vi "数据查询_仪器数据.vi"() -> ()   [LabVIEW 2016, in "数据查询.lvlib"]
uses:
  <vilib>/Utility/miscctls.llb/LVPointTypeDef.ctl
  <vilib>/Utility/miscctls.llb/LVRowAndColumnUnsignedTypeDef.ctl
  <userlib>/_OpenG.lib/array/array.llb/Sort 2D Array (String)__ogtk.vi
  <vilib>/ptbypt/NI_PtbyPt.lvlib
panel:
  out "布尔":bool=TRUE
  in  "显示关键参数":bool
  in  "剔除异常数据":bool
  in  "数据类型":string(combo)="全部数据"
  in  "列表框":i32(listbox)
  in  "页":i32 format="第%.0f页"
  in  "每页条数":i32=1000
  in  "向后按钮":bool
  in  "向前按钮":bool
  in  "导出":bool
  in  "测量模式":string(combo)="全部数据"
  in  "查询":bool
  in  "结束日期":string="2050/01/01"
  in  "起始日期":string="2010/01/01"
  out "数据表":string[][](table)
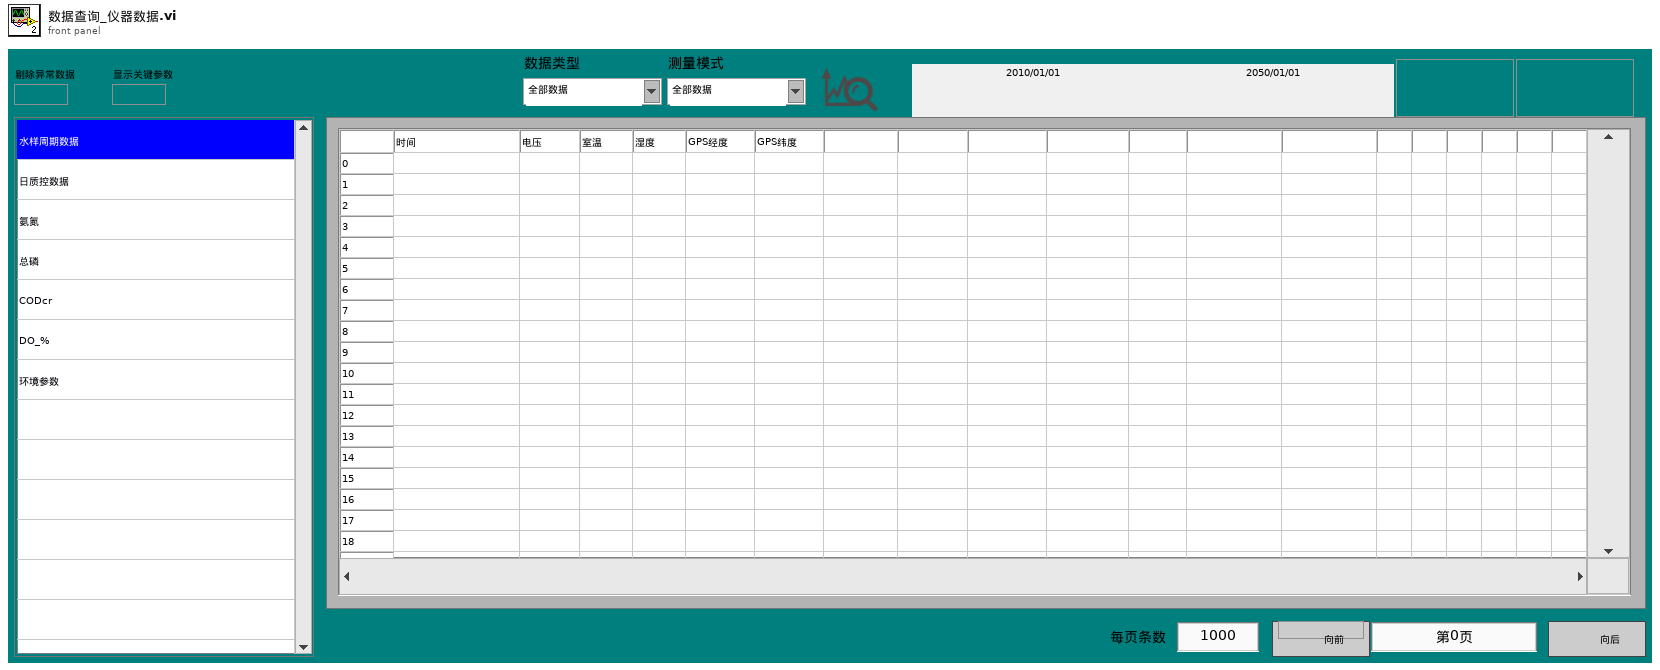
[diagram p1: front panel]
types:
  T1 = typedef "LVPointTypeDef.ctl" = cluster{"Horizontal":i16, "Vertical":i16}
  T2 = typedef "LVDateTimeRec.ctl" = cluster{"秒数的小数部分":dbl, "秒":i32, "分":i32, "时":i32, "日":i32, "月":i32, "年":i32, "天数（周）":i32, "天数（年）":i32, "DST":i32}
  T3 = typedef "Rendezvous RefNum" = refnum<k1>
  T4 = typedef "数据查询.lvlib/数据查询单选控件.ctl" = enum32{"数据查询", "仪器数据", "仪器日志", "报警信息", "校准日志"}
  T5 = enum8{"Enabled", "Disabled", "Disabled and Grayed Out"}
  T6 = typedef "LVRowAndColumnUnsignedTypeDef.ctl" = cluster{"Row":u32, "Column":u32}
  T7 = typedef "数据库类型.ctl" = enum16{"Access", "SQLite"}
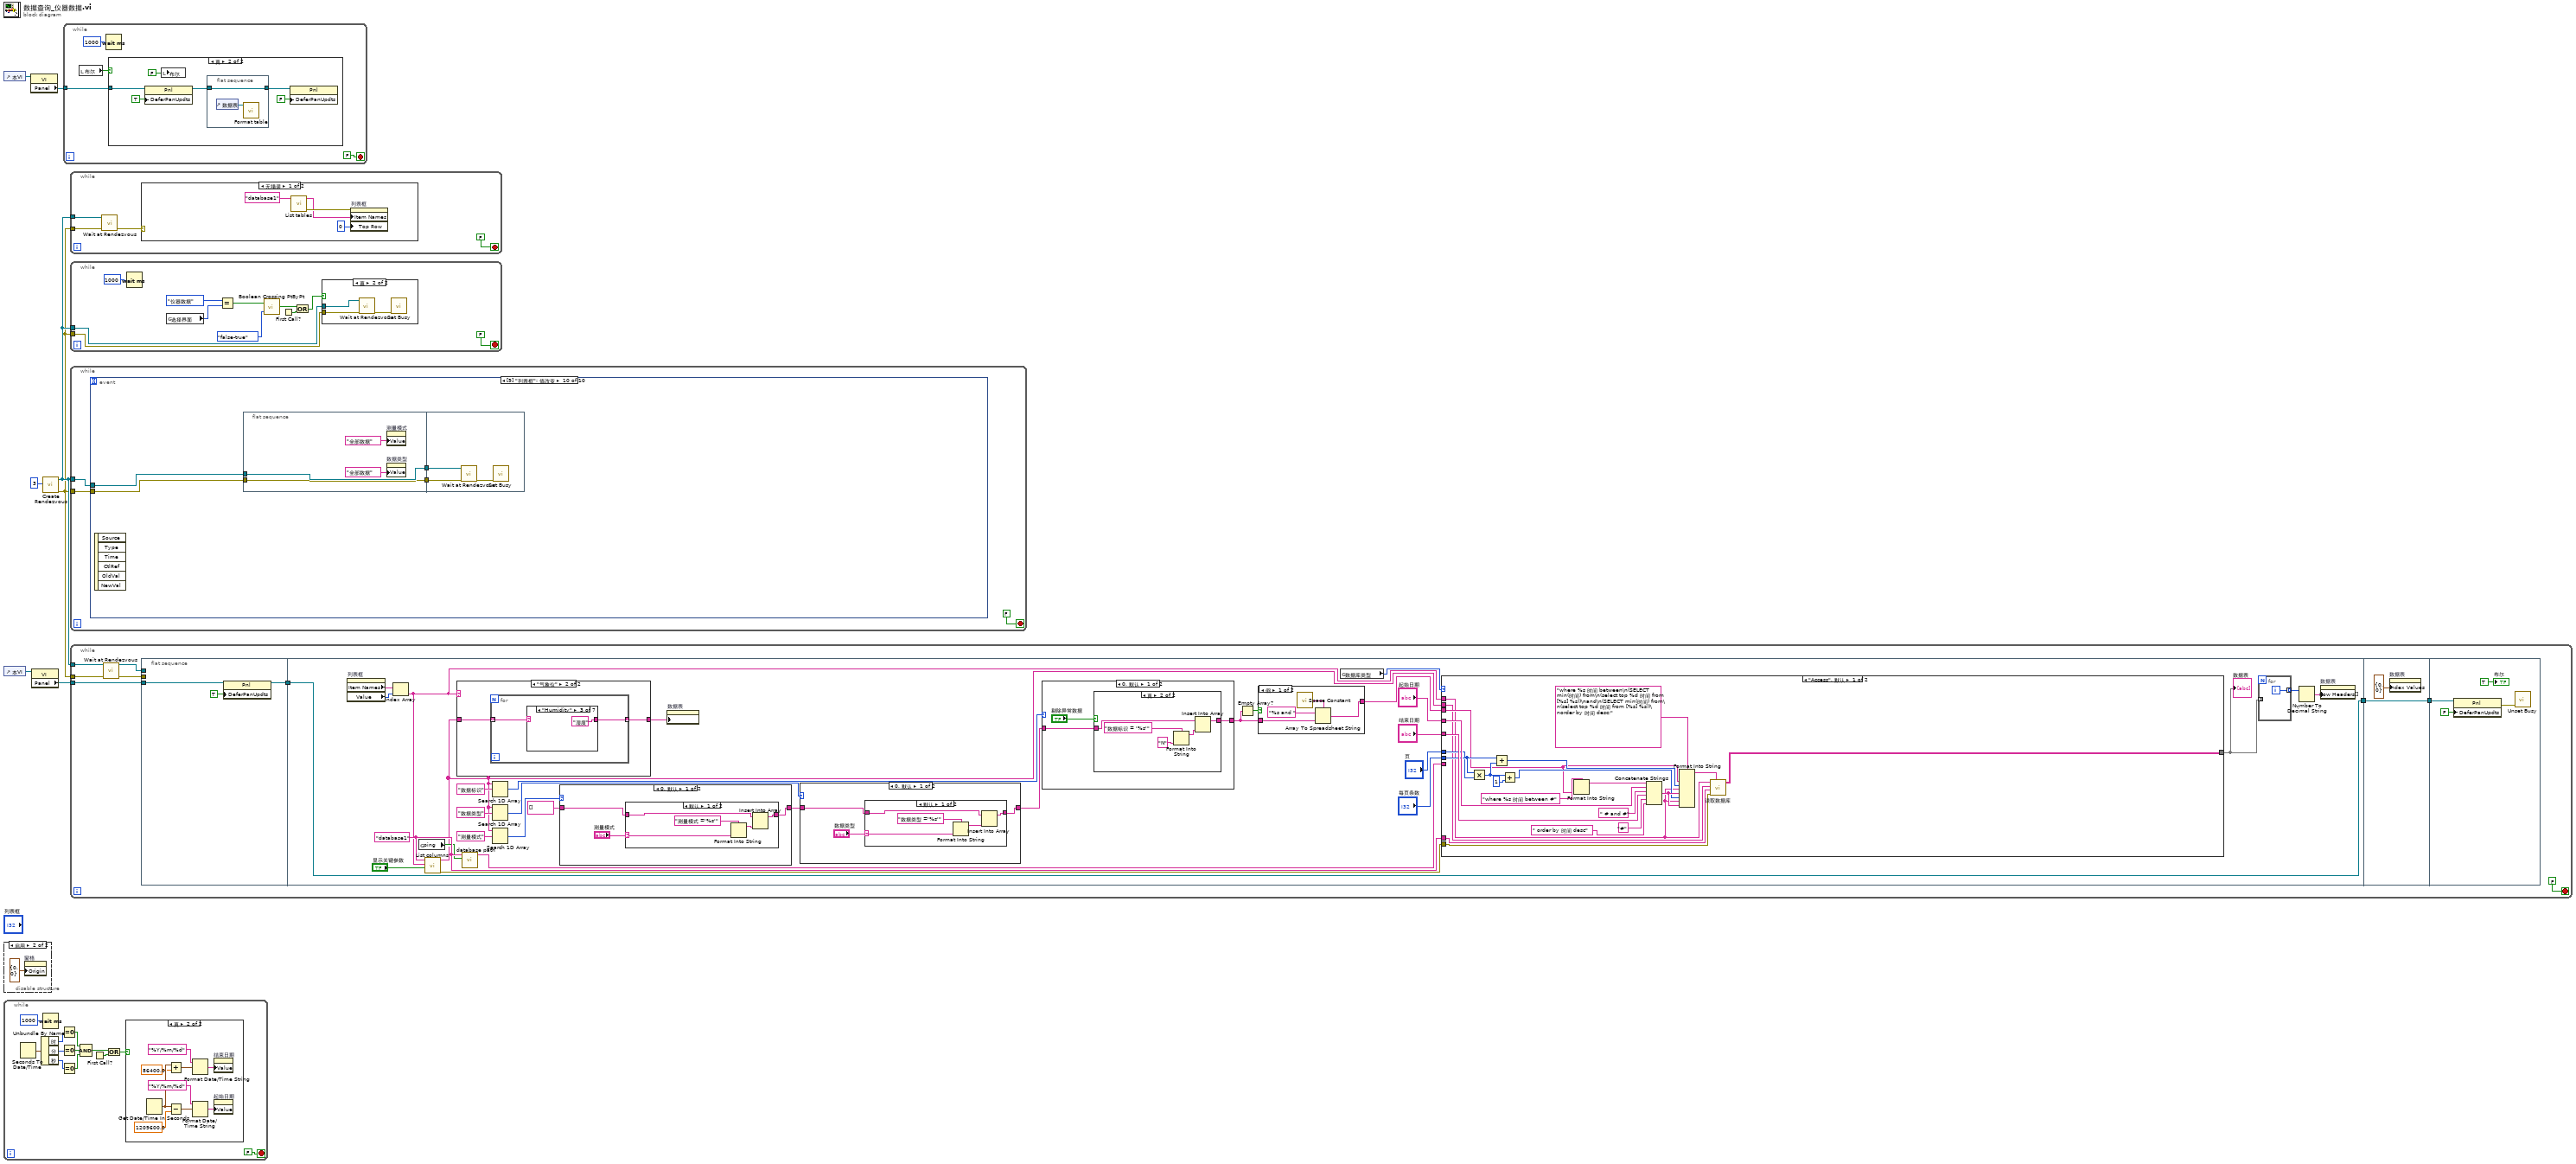
[diagram p0: block diagram]
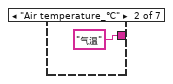
[diagram p7: hidden frame]
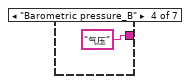
[diagram p8: hidden frame]
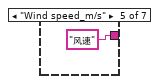
[diagram p9: hidden frame]
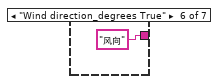
[diagram p10: hidden frame]
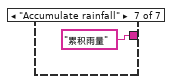
[diagram p11: hidden frame]
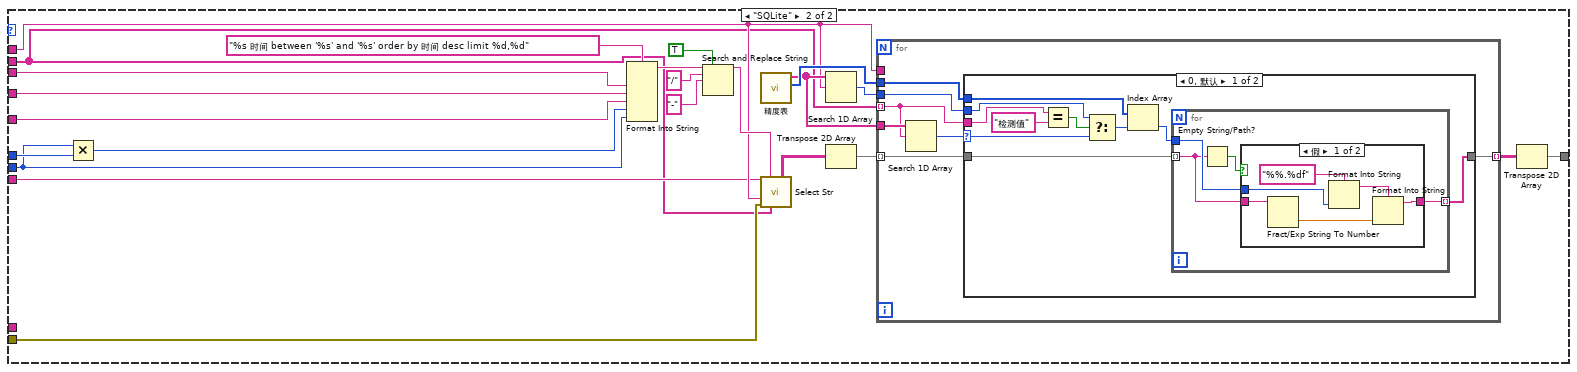
[diagram p12: hidden frame]
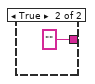
[diagram p15: hidden frame]
diagram:
  n1 = control-ref of="本VI"() -> (w4:refnum<vi>)
  n2 = control-ref of="本VI"() -> (w7:refnum<vi>)
  n3 = disable-structure shown="启用" {
    frame Disabled {
    }
    frame Enabled {
      n4 = property on="窗格" class="Pane"("Origin"=T1 {"Horizontal"=0, "Vertical"=0} ("原点")) -> ()  [unwired: 2 in, 2 out]
    }
  }
  n5 = while {
    stop <- FALSE stop-if-true
    n6 = Seconds To Date/Time() -> (date time rec=w20:T2)  [unwired: 2 in]
    n7 = Unbundle By Name(w20) -> ("时"=w19:i32, "分"=w18:i32, "秒"=w17:i32)
    n8 = Wait (ms)(milliseconds to wait=u32 1000 ("等待时间（毫秒）")) -> ()  [unwired: 1 out]
    n9 = Equal To 0?(x=w19) -> (x = 0?=w16:bool)
    n10 = Equal To 0?(x=w18) -> (x = 0?=w15:bool)
    n11 = Equal To 0?(x=w17) -> (x = 0?=w14:bool)
    n12 = Compound Arithmetic op=AND ("复合运算")(w16, w15, w14) -> (w11:bool)
    n13 = First Call?() -> (First Call?: T/F=w10:bool)
    n14 = Or(x=w11, y=w10) -> (x .or. y?=w9:bool)
    n15 = case shown="真" w9 {
      frame False {
      }
      frame True {
        n16 = Get Date/Time In Seconds() -> (seconds since 1Jan1904=w25:timestamp)
        n17 = Add(x=w25, y=86400.0) -> (x+y=w23:timestamp)
        n18 = Subtract(x=w25, y=1209600.0) -> (x-y=w26:timestamp)
        n19 = Format Date/Time String(time format string (%c)="%Y/%m/%d" ("时间格式字符串(%c)"), seconds (now)=w23) -> (date/time string=w22:string)  [unwired: 1 in]
        n20 = Format Date/Time String(time format string (%c)="%Y/%m/%d" ("时间格式字符串(%c)"), seconds (now)=w26) -> (date/time string=w28:string)  [unwired: 1 in]
        n21 = property on="结束日期" class="Str"("Value"=w22) -> ()  [unwired: 2 in, 2 out]
        n22 = property on="起始日期" class="Str"("Value"=w28) -> ()  [unwired: 2 in, 2 out]
      }
    }
  }
  n23 = property class="VI"(reference=w4) -> ("Panel"=w3:refnum<vi>)  [unwired: 1 in, 2 out]
  n24 = property class="VI"(reference=w7) -> ("Panel"=w6:refnum<vi>)  [unwired: 1 in, 2 out]
  n25 = call <vilib>:"Create Rendezvous.vi"("size (2)"=3) -> ("error out"=w1:errorcluster, "rendezvous"=w2:T3)  [unwired: 4 in, 1 out]
  n26 = while {
    tunnel: w3 -> [w32]
    stop <- FALSE stop-if-true
    n27 = local read "布尔"() -> (w31:bool)
    n28 = Wait (ms)(milliseconds to wait=u32 1000 ("等待时间（毫秒）")) -> ()  [unwired: 1 out]
    n29 = case shown="真" w31 {
      tunnel: w32 -> [_ w38]
      frame False {
      }
      frame True {
        n30 = property class="Pnl"(reference=w38, "DeferPanUpdts"=TRUE ("延迟前面板更新")) -> (reference out=w37:refnum<vi>)  [unwired: 1 in, 1 out]
        n31 = local write "布尔"(FALSE ("布尔")) -> ()
        n32 = flat-sequence {
          tunnel: [w41] -> w36
          tunnel: w37 -> [w41]
          frame #0 {
            n33 = control-ref of="数据表"() -> (w40:refnum<vi>)
            n34 = call "Format table.vi"("Table输入"=w40) -> ()  [unwired: 11 in]
          }
        }
        n35 = property class="Pnl"(reference=w36, "DeferPanUpdts"=FALSE ("延迟前面板更新")) -> ()  [unwired: 1 in, 2 out]
      }
    }
  }
  n36 = while {
    tunnel: w2 -> [w44]
    tunnel: w1 -> [w43]
    stop <- FALSE stop-if-true
    n37 = call <vilib>:"Wait at Rendezvous.vi"("error in (no error)"=w43, "rendezvous"=w44) -> ("error out"=w42:errorcluster)  [unwired: 3 in, 2 out]
    n38 = case shown="无错误" w42 {
      frame No Error {
        n39 = call "List tables.vi"("database"="database1") -> ("error out"=w49:errorcluster, "tables"=w46:string[])  [unwired: 9 in]
        n40 = property on="列表框" class="LstBox (严格)"(error in=w49, "Item Names"=w46, "Top Row"=0 ("顶行")) -> ()  [unwired: 1 in, 2 out]
      }
      frame Error {
      }
    }
  }
  n41 = while {
    tunnel: w2 -> [w51]
    tunnel: w1 -> [w50]
    stop <- FALSE stop-if-true
    n42 = Wait (ms)(milliseconds to wait=u32 1000 ("等待时间（毫秒）")) -> ()  [unwired: 1 out]
    n43 = global read "全局变量.vi" "选择界面"() -> (w58:T4)
    n44 = Equal?(x=数据查询单选控件."仪器数据", y=w58) -> (x = y?=w56:bool)
    n45 = call <vilib>:"Boolean Crossing PtByPt.vi"("direction"=enum16{"either", "false-true", "true-false"}."false-true", "input"=w56) -> ("crossing"=w54:bool)  [unwired: 1 in]
    n46 = First Call?() -> (First Call?: T/F=w52:bool)
    n47 = Or(x=w54, y=w52) -> (x .or. y?=w53:bool)
    n48 = case shown="真" w53 {
      tunnel: w51 -> [_ w63]
      tunnel: w50 -> [_ w62]
      frame False {
      }
      frame True {
        n49 = call <vilib>:"Wait at Rendezvous.vi"("error in (no error)"=w62, "rendezvous"=w63) -> ("error out"=w61:errorcluster)  [unwired: 3 in, 2 out]
        n50 = call <vilib>:"Set Busy.vi"("error in (no error)"=w61) -> ()  [unwired: 9 in, 2 out]
      }
    }
  }
  n51 = while {
    tunnel: w2 -> [w65]
    tunnel: w1 -> [w64]
    stop <- FALSE stop-if-true
    n52 = event shown="[9] \"列表框\": 值改变" {
      selector: _ -> [_ _ _ _ _ _ _ _ _ _]
      dyn-events: _ -> [_ _ _ _ _ _ _ _ _ _]
      timeout: _ -> [_ _ _ _ _ _ _ _ _ _]
      tunnel: w65 -> [_ _ _ _ _ _ _ _ w134 w138]
      tunnel: w64 -> [_ _ _ _ _ _ _ _ w133 w135]
      event Timeout {
        n53 = event-data() -> ()  [unwired: 1 in, 3 out]
      }
      event "查询": Mouse Down {
        n54 = event-data() -> ()  [unwired: 1 in, 8 out]
        n55 = property on="页" class="DigNum (严格)"("Value"=0 ("页")) -> ()  [unwired: 2 in, 2 out]
      }
      event "每页条数": Mouse Down {
        n56 = event-data() -> ("CtlRef"=w69:refnum<vi>)  [unwired: 1 in, 7 out]
        n57 = property class="DigNum (严格)"(reference=w69) -> (reference out=w70:refnum<vi>, "Value"=w72:i32)  [unwired: 1 in, 1 out]
        n58 = property on="页" class="DigNum (严格)"("Value"=0 ("页")) -> ()  [unwired: 2 in, 2 out]
        n59 = call "数字键盘.vi"("OldNumber"=w72) -> ("NewNumber"=w71:sgl)
        n60 = property class="DigNum (严格)"(reference=w70, "Val(Sgnl)"=w71) -> ()  [unwired: 1 in, 2 out]
      }
      event "页": Mouse Down {
        n61 = event-data() -> ("CtlRef"=w73:refnum<vi>)  [unwired: 1 in, 7 out]
        n62 = property class="DigNum (严格)"(reference=w73) -> (reference out=w74:refnum<vi>, "Value"=w76:i32)  [unwired: 1 in, 1 out]
        n63 = call "数字键盘.vi"("OldNumber"=w76) -> ("NewNumber"=w75:sgl)
        n64 = property class="DigNum (严格)"(reference=w74, "Val(Sgnl)"=w75) -> ()  [unwired: 1 in, 2 out]
      }
      event "向前按钮": Value Change {
        n65 = event-data() -> ()  [unwired: 1 in, 6 out]
        n66 = property on="页" class="DigNum (严格)"() -> ("Value"=w82:i32)  [unwired: 2 in, 2 out]
        n67 = Decrement(x=w82) -> (x-1=w81:i32)
        n68 = In Range and Coerce(upper limit=9999 ("上限"), x=w81, lower limit=0 ("下限")) -> (coerced(x)=w78:i32, In Range?=w77:bool)
        n69 = case shown="真" w77 {
          tunnel: w78 -> [_ w83]
          frame False {
          }
          frame True {
            n70 = property on="页" class="DigNum (严格)"("Val(Sgnl)"=w83) -> ()  [unwired: 2 in, 2 out]
          }
        }
      }
      event "向后按钮": Value Change {
        n71 = event-data() -> ()  [unwired: 1 in, 6 out]
        n72 = property on="页" class="DigNum (严格)"() -> ("Value"=w88:i32)  [unwired: 2 in, 2 out]
        n73 = Increment(x=w88) -> (x+1=w87:i32)
        n74 = In Range and Coerce(upper limit=u32 9999 ("上限"), x=w87, lower limit=u32 0 ("下限")) -> (coerced(x)=w84:u32)  [unwired: 1 out]
        n75 = property on="页" class="DigNum (严格)"("Val(Sgnl)"=w84) -> ()  [unwired: 2 in, 2 out]
      }
      event "导出": Value Change {
        n76 = event-data() -> ("CtlRef"=w89:refnum<vi>)  [unwired: 1 in, 5 out]
        n77 = property class="Bool"(reference=w89, "DisabledEnum"=T5."Disabled and Grayed Out" ("禁用")) -> (reference out=w93:refnum<vi>, error out=w94:errorcluster)  [unwired: 1 in]
        n78 = flat-sequence {
          tunnel: w94 -> [_]
          tunnel: [w113] -> w92
          tunnel: w93 -> [w113]
          tunnel: "导出" -> [_]
          frame #0 {
            n79 = local read "数据表"() -> (w117:string[][])
            n80 = call-poly <userlib>:"Sort Array__ogtk.vi"("Column/Row to Sort By"=u32 0, "Sort By in"=enum16{"row", "column"}."column", "Order"=enum16{"ascending", "descending"}."ascending", "Array in"=w117) -> ("Sorted Array out"=w99:string[][])  [unwired: 4 in, 3 out]
            n81 = for {
              tunnel: w99 -> [w126] mode=indexing
              tunnel: [w125] -> w103 mode=indexing
              i -> [w127]
              n82 = Increment(x=w127) -> (x+1=w123:i32)
              n83 = Number To Decimal String(number=w123) -> (decimal integer string=w122:string)  [unwired: 1 in]
              n84 = Insert Into Array(array=w126, index=0 ("索引"), new element=w122) -> (w125:string[])
            }
            n85 = property on="数据表" class="Tbl (严格)"() -> ("Column Headers[]"=w106:string[])  [unwired: 2 in, 2 out]
            n86 = property on="列表框" class="LstBox (严格)"() -> ("Item Names"=w98:string[], "Value"=w97:i32)  [unwired: 2 in, 2 out]
            n87 = Insert Into Array(array=w106, index=0 ("索引"), new element="序号" ("新元素/子数组")) -> (w107:string[])
            n88 = Index Array(array=w98, index=w97) -> (element=w96:string)
            n89 = Format Date/Time String(time format string (%c)="%y_%m_%d" ("时间格式字符串(%c)")) -> (date/time string=w110:string)  [unwired: 2 in]
            n90 = Concatenate Strings(w96, "_" ("字符串"), w110) -> (w108:string)
            n91 = Insert Into Array(array=string[][] [], new element #1=w107, new element #2=w103) -> (w102:string[][])  [unwired: 2 in]
            n92 = call "数据导出Excel.vi"("text data"=w102, "default name"=w108) -> ("error out"=w101:errorcluster, "布尔"=w100:bool)  [unwired: 8 in]
            n93 = case shown="真" w100 {
              tunnel: w101 -> [_ w119]
              frame False {
              }
              frame True {
                n94 = case shown="错误" w119 {
                  tunnel: ["导出成功" ("消息") "导出失败" ("消息")] -> w118
                  frame No Error {
                  }
                  frame Error {
                  }
                }
                n95 = One Button Dialog(message=w118) -> ()  [unwired: 1 in, 1 out]
              }
            }
          }
        }
        n96 = property class="Bool"(reference=w92, "DisabledEnum"=T5."Enabled" ("禁用")) -> ()  [unwired: 1 in, 2 out]
      }
      event "起始日期", "结束日期": Mouse Down {
        n97 = event-data() -> ("CtlRef"=w131:refnum<vi>)  [unwired: 1 in, 7 out]
        n98 = property class="Str"(reference=w131) -> (reference out=w129:refnum<vi>, "Value"=w130:string)  [unwired: 1 in, 1 out]
        n99 = call "日期键盘.vi"("原值"=w130) -> ("x+y"=w128:string)  [unwired: 10 in]
        n100 = property class="Str"(reference=w129, "Val(Sgnl)"=w128) -> ()  [unwired: 1 in, 2 out]
      }
      event "查询", "起始日期", "结束日期", "测量模式", "页", "每页条数", "数据类型", "剔除异常数据": Value Change {
        n101 = event-data() -> ()  [unwired: 1 in, 6 out]
        n102 = call <vilib>:"Wait at Rendezvous.vi"("error in (no error)"=w133, "rendezvous"=w134) -> ("error out"=w132:errorcluster)  [unwired: 3 in, 2 out]
        n103 = call <vilib>:"Set Busy.vi"("error in (no error)"=w132) -> ()  [unwired: 9 in, 2 out]
      }
      event "列表框": Value Change {
        n104 = event-data() -> ()  [unwired: 1 in, 6 out]
        n105 = flat-sequence {
          tunnel: w138 -> [w142]
          tunnel: [w142] -> w137
          tunnel: [w139] -> w136
          tunnel: w135 -> [w139]
          tunnel: w137 -> [w145]
          tunnel: w136 -> [w144]
          frame #0 {
            n106 = property on="测量模式" class="CmbBox"("Value"="全部数据" ("测量模式")) -> ()  [unwired: 2 in, 2 out]
            n107 = property on="数据类型" class="CmbBox"("Value"="全部数据" ("数据类型")) -> ()  [unwired: 2 in, 2 out]
          }
          frame #1 {
            n108 = call <vilib>:"Wait at Rendezvous.vi"("error in (no error)"=w144, "rendezvous"=w145) -> ("error out"=w143:errorcluster)  [unwired: 3 in, 2 out]
            n109 = call <vilib>:"Set Busy.vi"("error in (no error)"=w143) -> ()  [unwired: 9 in, 2 out]
          }
        }
      }
    }
  }
  n110 = while {
    tunnel: w2 -> [w149]
    tunnel: w6 -> [w153]
    tunnel: w1 -> [w148]
    stop <- FALSE stop-if-true
    n111 = call <vilib>:"Wait at Rendezvous.vi"("error in (no error)"=w148, "rendezvous"=w149) -> ("error out"=w146:errorcluster, "rendezvous out"=w147:T3)  [unwired: 3 in, 1 out]
    n112 = flat-sequence {
      tunnel: w153 -> [w157]
      tunnel: [w155] -> w152
      tunnel: w147 -> [_]
      tunnel: w146 -> [_]
      tunnel: w152 -> [w158]
      tunnel: [w158] -> w150
      tunnel: [w311] -> w151
      tunnel: w150 -> [w311]
      tunnel: w151 -> [w316]
      frame #0 {
        n113 = property class="Pnl"(reference=w157, "DeferPanUpdts"=TRUE ("延迟前面板更新")) -> (reference out=w155:refnum<vi>)  [unwired: 1 in, 1 out]
      }
      frame #1 {
        w166 = "database1" ("database")
        n114 = property on="列表框" class="LstBox (严格)"() -> ("Item Names"=w177:string[], "Value"=w182:i32)  [unwired: 2 in, 2 out]
        n115 = Index Array(array=w177, index=w182) -> (element=w161:string)
        n116 = global read "全局变量.vi" "ping"() -> (w164:bool)
        n117 = call "List columns.vi"("显示关键参数"="显示关键参数", "table"=w161, "database"=w166) -> ("error out"=w176:errorcluster, "columns"=w162:string[])  [unwired: 7 in]
        n118 = case shown="\"气象仪\"" w161 {
          tunnel: w162 -> [w189 w191]
          tunnel: [w189 w190] -> w160
          frame "假", Default {
          }
          frame "气象仪" {
            n119 = for {
              tunnel: w191 -> [w193] mode=indexing
              tunnel: [w192] -> w190 mode=indexing
              n120 = case shown="\"Humidity\"" w193 {
                selector: w193 -> [w194 _ _ _ _ _ _]
                tunnel: [w194 "气温" "湿度" "气压" "风速" "风向" "累积雨量"] -> w192
                frame "", Default {
                }
                frame "Air temperature_℃" {
                }
                frame "Humidity" {
                }
                frame "Barometric pressure_B" {
                }
                frame "Wind speed_m/s" {
                }
                frame "Wind direction_degrees True" {
                }
                frame "Accumulate rainfall" {
                }
              }
            }
          }
        }
        n121 = call "database path.vi"("ping"=w164, "database"=w166) -> ("Path out"=w165:string)  [unwired: 8 in, 1 out]
        n122 = Search 1D Array(1D array=w162, element="数据标识" ("元素")) -> (index of element=w171:i32)  [unwired: 1 in]
        n123 = Search 1D Array(1D array=w162, element="数据类型" ("元素")) -> (index of element=w173:i32)  [unwired: 1 in]
        n124 = Search 1D Array(1D array=w162, element="测量模式" ("元素")) -> (index of element=w170:i32)  [unwired: 1 in]
        n125 = case shown="0, 默认" w170 {
          tunnel: string[] [] -> [w282 w289]
          tunnel: [w280 w289] -> w179
          frame 0, Default {
            n126 = case shown="默认" "测量模式" {
              selector: "测量模式" -> [w283 _]
              tunnel: w282 -> [w286 w288]
              tunnel: [w284 w288] -> w280
              frame Default {
                n127 = Format Into String(format string="测量模式 ='%s'" ("condition"), w283) -> (resulting string=w285:string)  [unwired: 2 in, 1 out]
                n128 = Insert Into Array(array=w286, new element=w285) -> (w284:string[])  [unwired: 1 in]
              }
              frame "全部数据" {
              }
            }
          }
          frame -1 {
          }
        }
        n129 = property on="数据表" class="Tbl (严格)"("Column Headers[]"=w160) -> ()  [unwired: 2 in, 2 out]
        n130 = case shown="0, 默认" w173 {
          tunnel: w179 -> [w302 w309]
          tunnel: [w301 w309] -> w175
          frame 0, Default {
            n131 = case shown="默认" "数据类型" {
              selector: "数据类型" -> [w303 _]
              tunnel: w302 -> [w306 w308]
              tunnel: [w304 w308] -> w301
              frame Default {
                n132 = Format Into String(format string="数据类型 ='%s'" ("condition"), w303) -> (resulting string=w305:string)  [unwired: 2 in, 1 out]
                n133 = Insert Into Array(array=w306, new element=w305) -> (w304:string[])  [unwired: 1 in]
              }
              frame "全部数据" {
              }
            }
          }
          frame -1 {
          }
        }
        n134 = case shown="0, 默认" w171 {
          tunnel: [w292 w299] -> w168
          tunnel: w175 -> [w290 w299]
          frame 0, Default {
            n135 = case shown="真" "剔除异常数据" {
              tunnel: w290 -> [w293 w298]
              tunnel: [w293 w297] -> w292
              frame False {
              }
              frame True {
                n136 = Format Into String(format string="数据标识 = '%s'" ("condition"), "N" ("String")) -> (resulting string=w294:string)  [unwired: 2 in, 1 out]
                n137 = Insert Into Array(array=w298, new element=w294) -> (w297:string[])  [unwired: 1 in]
              }
            }
          }
          frame -1 {
          }
        }
        n138 = Empty Array?(array=w168) -> (empty?=w167:bool)
        n139 = case shown="假" w167 {
          tunnel: [w276 "" ("spreadsheet string")] -> w178
          tunnel: w168 -> [w275 _]
          frame False {
            n140 = call <vilib>:"Space Constant.vi"() -> ("String"=w278:string)
            n141 = Array To Spreadsheet String(delimiter (Tab)=w278, array=w275, 3:"%s and " ("格式字符串")) -> (spreadsheet string=w276:string)
          }
          frame True {
          }
        }
        n142 = global read "外部调用接口全局变量.vi" "数据库类型"() -> (w159:T7)
        n143 = case shown="\"Access\", 默认" w159 {
          tunnel: "起始日期" -> [w222 w242]
          tunnel: "结束日期" -> [w221 w241]
          tunnel: "每页条数" -> [w214 w239]
          tunnel: "页" -> [w213 w240]
          tunnel: [w212 w229] -> w181
          tunnel: w178 -> [w205 w243]
          tunnel: w176 -> [w204 w245]
          tunnel: w161 -> [w203 w226]
          tunnel: w166 -> [w202 _]
          tunnel: w162 -> [w201 w223]
          tunnel: w165 -> [_ w224]
          frame "Access", Default {
            n144 = Multiply(x=w214, y=w213) -> (x*y=w210:i32)
            n145 = Add(x=w214, y=w210) -> (x+y=w208:i32)
            n146 = Add(x=w210, y=u32 1) -> (x+y=w207:u32)
            n147 = Format Into String(format string="where %s 时间 between #" ("condition"), w205) -> (resulting string=w218:string)  [unwired: 2 in, 1 out]
            n148 = Concatenate Strings(w218, w222, " # and #" ("condition"), w221, "#" ("condition"), " order by 时间 desc" ("字符串")) -> (w216:string)
            n149 = Format Into String(format string="where %s 时间 between\n(SELECT min(时间) from\n(select top %d 时间 from [%s] %s))\nand\n(SELECT min(时间) from\n(select top %d 时间 from [%s] %s))\norder by 时间 desc;" ("格式字符串"), w205, w208, w203, w216, w207, w203, w216) -> (resulting string=w215:string)  [unwired: 2 in, 1 out]
            n150 = call "读取数据库.vi"("condition"=w215, "error in (no error)"=w204, "database"=w202, "显示项"=w201, "组合框"=w203) -> ("表格"=w212:string[][])  [unwired: 3 in, 3 out]
          }
          frame "SQLite" {
            n151 = Multiply(x=w239, y=w240) -> (x*y=w238:i32)
            n152 = Format Into String(format string="%s 时间 between '%s' and '%s' order by 时间 desc limit %d,%d" ("格式字符串"), w243, w242, w241, w238, w239) -> (resulting string=w234:string)  [unwired: 2 in, 1 out]
            n153 = Search and Replace String(replace all?=TRUE ("替换全部？(F)"), input string=w234, search string="/" ("搜索字符串"), replace string="-" ("替换字符串(\"\")")) -> (result string=w233:string)  [unwired: 4 in, 3 out]
            n154 = call "精度表.vi"() -> ("精度"=w228:i32[], "参数"=w227:string[])  [unwired: 10 in]
            n155 = call "Select Str.vi"("DB Path"=w224, "Where Clause"=w233, "Tables Name"=w226, "error in (no error)"=w245, "Columns"=w223) -> ("Results"=w232:string[][])  [unwired: 7 in, 3 out]
            n156 = Search 1D Array(1D array=w227, element=w226) -> (index of element=w225:i32)  [unwired: 1 in]
            n157 = Transpose 2D Array(2D array=w232) -> (transposed array=w231:string[][])
            n158 = for {
              tunnel: w223 -> [w247] mode=indexing
              tunnel: w231 -> [w252] mode=indexing
              tunnel: [w251] -> w230 mode=indexing
              tunnel: w226 -> [_]
              tunnel: w227 -> [w248]
              tunnel: w228 -> [w250]
              tunnel: w225 -> [w246]
              n159 = Search 1D Array(1D array=w248, element=w247) -> (index of element=w249:i32)  [unwired: 1 in]
              n160 = case shown="0, 默认" w249 {
                selector: w249 -> [w254 _]
                tunnel: w252 -> [w262 w274]
                tunnel: [w261 w274] -> w251
                tunnel: w250 -> [w260 _]
                tunnel: w247 -> [w257 _]
                tunnel: w246 -> [w255 _]
                frame 0, Default {
                  n161 = Equal?(x=w257, y="检测值" ("元素")) -> (x = y?=w256:bool)
                  n162 = Select(t=w255, s=w256, f=w254) -> (s? t:f=w253:i32)
                  n163 = Index Array(array=w260, index=w253) -> (element=w259:i32)
                  n164 = for {
                    tunnel: w262 -> [w264] mode=indexing
                    tunnel: [w265] -> w261 mode=indexing
                    tunnel: w259 -> [w266]
                    n165 = Empty String/Path?(string/path=w264) -> (empty?=w263:bool)
                    n166 = case shown="假" w263 {
                      tunnel: w266 -> [w271 _]
                      tunnel: [w268 w273] -> w265
                      tunnel: w264 -> [w267 w273]
                      frame False {
                        n167 = Fract/Exp String To Number(string=w267) -> (number=w272:dbl)  [unwired: 3 in, 1 out]
                        n168 = Format Into String(format string="%%.%df" ("格式字符串"), w271) -> (resulting string=w270:string)  [unwired: 2 in, 1 out]
                        n169 = Format Into String(format string=w270, w272) -> (resulting string=w268:string)  [unwired: 2 in, 1 out]
                      }
                      frame True {
                      }
                    }
                  }
                }
                frame -1 {
                }
              }
            }
            n170 = Transpose 2D Array(2D array=w230) -> (transposed array=w229:string[][])
          }
        }
        "数据表" <- w181
        n171 = for {
          tunnel: w181 -> [_] mode=indexing
          tunnel: [w310] -> w186 mode=indexing
          i -> [w310]
        }
        n172 = Number To Decimal String(number=w186) -> (decimal integer string=w185:string[])  [unwired: 1 in]
        n173 = property on="数据表" class="Tbl (严格)"("Row Headers[]"=w185) -> ()  [unwired: 2 in, 2 out]
      }
      frame #2 {
        n174 = property on="数据表" class="Tbl (严格)"("Index Values"=T6 {"Row"=0, "Column"=0} ("索引值")) -> ()  [unwired: 2 in, 2 out]
      }
      frame #3 {
        n175 = property class="Pnl"(reference=w316, "DeferPanUpdts"=FALSE ("延迟前面板更新")) -> (error out=w314:errorcluster)  [unwired: 1 in, 1 out]
        n176 = call <vilib>:"Unset Busy.vi"("error in (no error)"=w314) -> ()  [unwired: 10 in, 1 out]
        "布尔" <- TRUE
      }
    }
  }
